vi "csvCleaner.vi"(8 "error in (no error)":errorcluster, 9 "FIFO Garbage Start (1)":i32=1, 10 "FIFO Garbage Length (5)":i32=5, 11 "CSV Input File":path) -> (0 "error out":errorcluster, 1 "Clean":string[][](array[string]), 2 "Clean+No Dups":string[][](array[string]), 3 "CSV Output File":path, 4 "Clean Dups Size":i32[](array[numeric]), 5 "all rows":string[][](array[string]), 6 "Clean FIFO Size":i32[](array[numeric]))   [LabVIEW 2019]
uses:
  <vilib>/Utility/file.llb/Read Delimited Spreadsheet (string).vi
  1df47058-c119-4b07-bab9-3d180fa7a268.vi
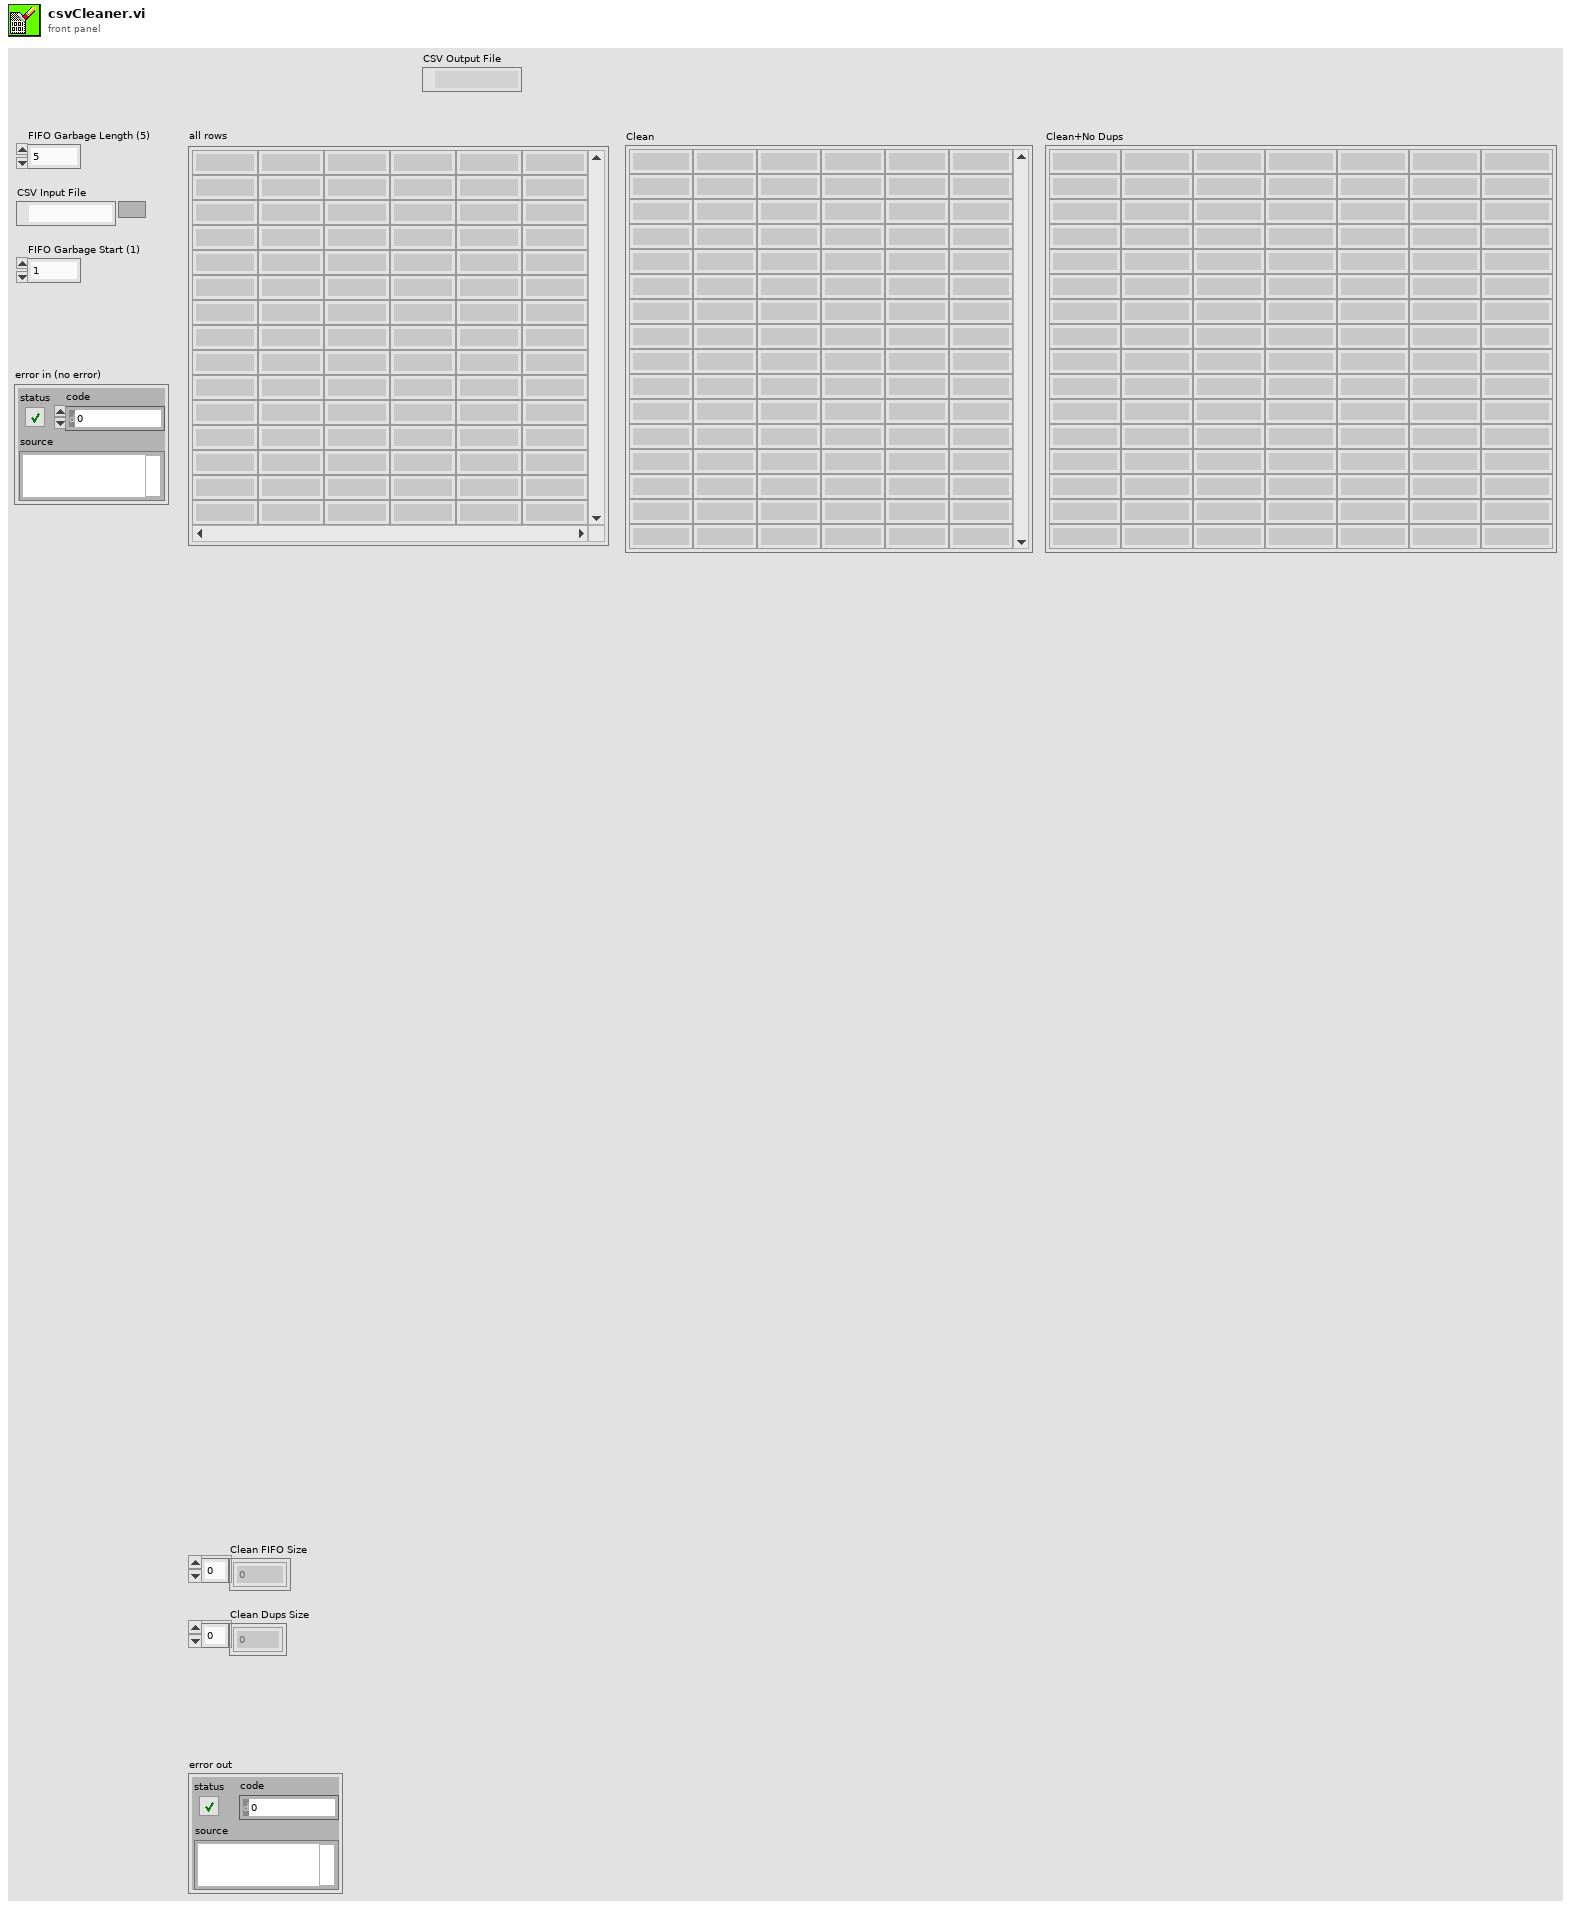
[diagram p1: front panel]
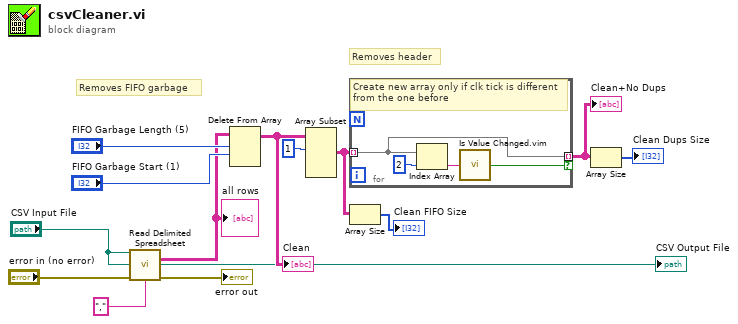
[diagram p0: block diagram]
diagram:
  # "Removes FIFO garbage"
  # "Removes header"
  n1 = call-poly <vilib>:"Read Delimited Spreadsheet.vi"("file path (dialog if empty)"="CSV Input File", "error in (no error)"="error in (no error)", "delimiter (\\t)"=",") -> ("all rows"=w6:string[][], "error out"=→"error out":errorcluster)  [unwired: 7 in, 4 out]
  "all rows" <- w6
  n2 = Delete From Array(array=w6, length="FIFO Garbage Length (5)", index (row)="FIFO Garbage Start (1)") -> (array with subset deleted=w9:string[][])  [unwired: 1 in, 1 out]
  "Clean" <- w9
  n3 = Array Subset(array=w9, index (row)=1 ("index")) -> (w13:string[][])  [unwired: 3 in]
  n4 = for {
    tunnel: [w14] -> w10 mode=indexing if=w15
    tunnel: w13 -> [w14] mode=indexing
    # "Create new array only if clk tick is different from the one before"
    n5 = Index Array(array=w14, index=2) -> (element=w16:string)
    n6 = call "Is Value Changed.vim"("value"=w16) -> ("changed or first call?"=w15:bool)
  }
  "Clean+No Dups" <- w10
  n7 = Array Size(array=w13) -> (size(s)=→"Clean FIFO Size":i32[])
  n8 = Array Size(array=w10) -> (size(s)=→"Clean Dups Size":i32[])
  "CSV Output File" <- "CSV Input File"
